vi "Enhance niSync Error.vi"(6 "sync config label":string="Time-Based Synchronization Module name", 8 "error in (no error)":errorcluster, 10 "custom device name":string="NI Synchronization", 11 "resource name":string) -> (0 "error out":errorcluster)   [LabVIEW 2015, in "NI Synchronization Engine.lvlib"]
uses:
  NI Synchronization Engine.lvlib
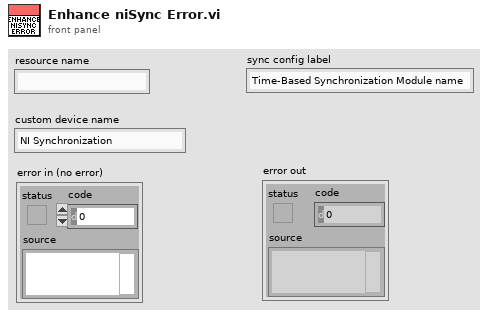
[diagram p1: front panel]
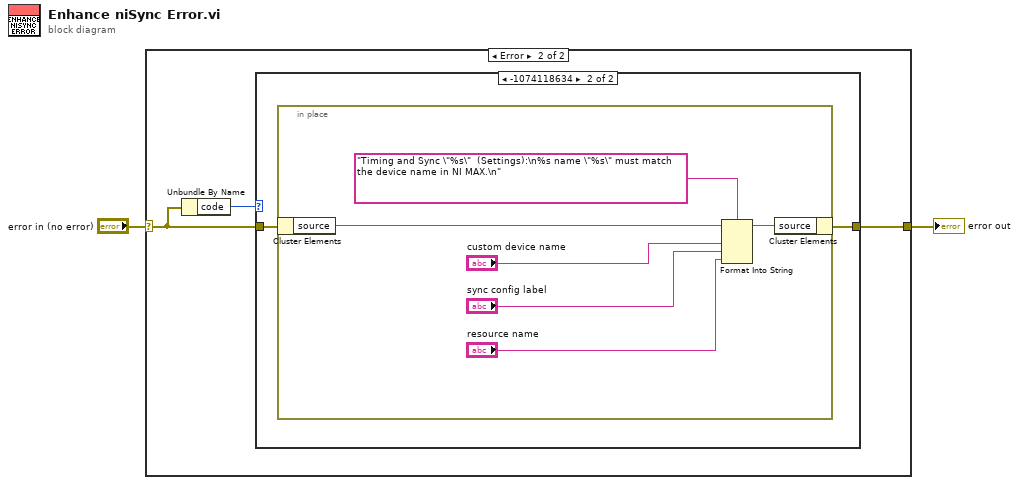
[diagram p0: block diagram]
diagram:
  n1 = case shown="Error" "error in (no error)" {
    selector: "error in (no error)" -> [w3 w6]
    tunnel: [w3 w5] -> w2
    frame No Error {
    }
    frame Error {
      n2 = Unbundle By Name(w6) -> ("code"=w4:i32)
      n3 = case shown="-1074118634" w4 {
        tunnel: [w7 w8] -> w5
        tunnel: w6 -> [w7 w9]
        frame Default {
        }
        frame -1074118634 {
          n4 = in-place {
            n5 = in-place-cluster #1(w9) -> ("source"=w12:string)
            n6 = Format Into String(format string="Timing and Sync \"%s\"  (Settings):\n%s name \"%s\" must match the device name in NI MAX.\n", initial string=w12, "custom device name", "sync config label", "resource name") -> (resulting string=w11:string)  [unwired: 1 in, 1 out]
            n7 = in-place-cluster #1("source"=w11) -> (w8:errorcluster)
          }
        }
      }
    }
  }
  "error out" <- w2
